vi "Trim stitching data.vi"() -> ()   [LabVIEW 2017]
panel:
  out "Deleting...":path
  in  "Path":path=path "C:/Users/Theo/Desktop/RAW (trimmed down)"
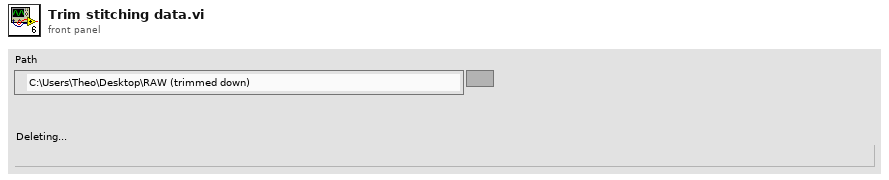
[diagram p1: front panel]
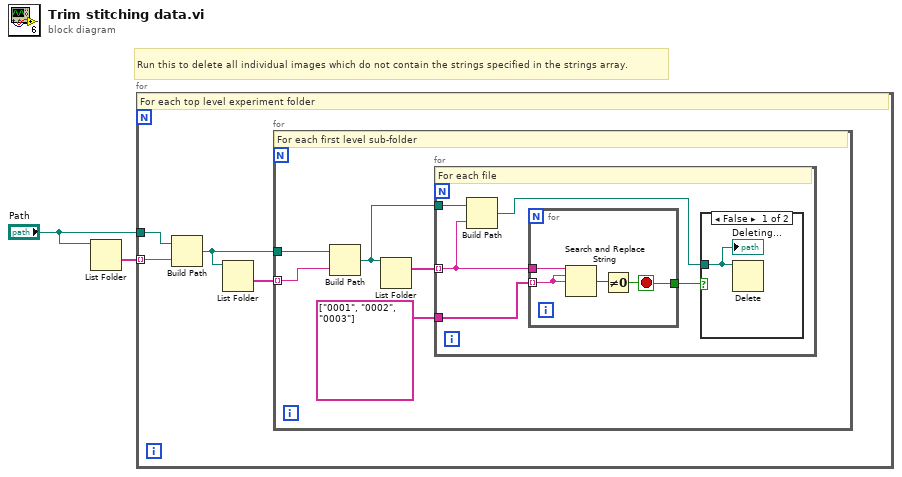
[diagram p0: block diagram]
diagram:
  # "Run this to delete all individual images which do not contain the strings specified in the strings array."
  n1 = List Folder(path="Path") -> (folder names=w2:string[])  [unwired: 3 in, 3 out]
  n2 = for {
    tunnel: w2 -> [w6] mode=indexing
    tunnel: "Path" -> [w5]
    # "For each top level experiment folder"
    n3 = Build Path(base path=w5, name or relative path=w6) -> (appended path=w4:path)
    n4 = List Folder(path=w4) -> (folder names=w3:string[])  [unwired: 3 in, 3 out]
    n5 = for {
      tunnel: w4 -> [w8]
      tunnel: w3 -> [w7] mode=indexing
      # "For each first level sub-folder"
      n6 = Build Path(base path=w8, name or relative path=w7) -> (appended path=w11:path)
      n7 = List Folder(path=w11) -> (filenames=w10:string[])  [unwired: 3 in, 3 out]
      n8 = for {
        tunnel: w11 -> [w16]
        tunnel: w10 -> [w15] mode=indexing
        tunnel: string[] ["0001", "0002", "0003"] -> [w14]
        # "For each file"
        n9 = Build Path(base path=w16, name or relative path=w15) -> (appended path=w12:path)
        n10 = for {
          tunnel: w15 -> [w21]
          tunnel: w14 -> [w20] mode=indexing
          tunnel: [w18] -> w13
          stop <- w18 stop-if-true
          n11 = Search and Replace String(input string=w21, search string=w20, replace string=w20) -> (number of replacements=w19:i32)  [unwired: 5 in, 3 out]
          n12 = Not Equal To 0?(x=w19) -> (x != 0?=w18:bool)
        }
        n13 = case shown="False" w13 {
          tunnel: w12 -> [w17 _]
          frame False {
            n14 = Delete(path (use dialog)=w17) -> ()  [unwired: 4 in, 3 out]
            "Deleting..." <- w17
          }
          frame True {
          }
        }
      }
    }
  }
